vi "Resize Pane.vi"(6 "Pane size":i32, 8 "error in (no error)":errorcluster, 11 "Splitter in":refnum<class "Splitter.lvclass">) -> (0 "error out":errorcluster, 2 "Resized?":bool, 3 "Splitter out":refnum<class "Splitter.lvclass">)   [LabVIEW 2021, in "Splitter.lvclass"]
doc: "Copyright 2018, Wiebe Walstra, wiebe@carya.nl."
uses:
  Splitter.lvclass
  C:/Projects/Dynamic-Scaling/Dynamic Scaling/IContainer/Divider/Divider.lvclass
  Splitter.lvclass/Splitter.ctl
  Divider.lvclass
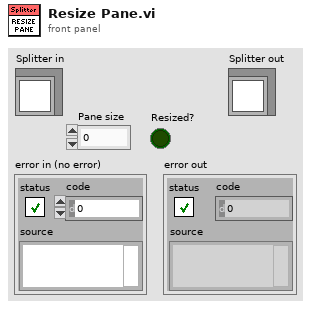
[diagram p1: front panel]
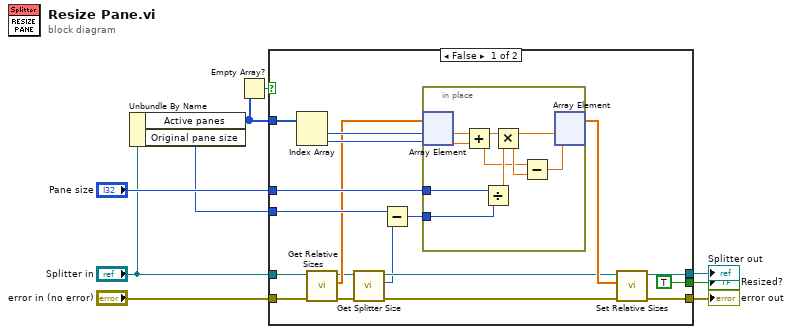
[diagram p0: block diagram]
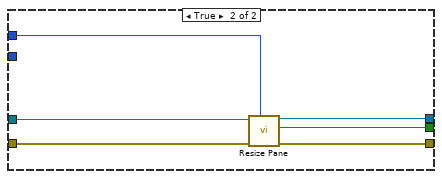
[diagram p2: hidden frame]
diagram:
  n1 = Unbundle By Name("Splitter in") -> ("Active panes"=w2:i32[], "Original pane size"=w1:i16)
  n2 = Empty Array?(array=w2) -> (empty?=w3:bool)
  n3 = case shown="False" w3 {
    tunnel: [w16 w41] -> w9
    tunnel: [TRUE ("Resized?") w40] -> w8
    tunnel: [w14 w39] -> w7
    tunnel: "Pane size" -> [w25 w38]
    tunnel: "error in (no error)" -> [w26 w37]
    tunnel: "Splitter in" -> [w18 w36]
    tunnel: w2 -> [w24 _]
    tunnel: w1 -> [w23 _]
    frame False {
      n4 = Index Array(array=w24) -> (element #1=w22:i32, element #2=w21:i32)  [unwired: 2 in]
      n5 = call "Get Relative Sizes.vi"("error in (no error)"=w26, "Divider in"=w18) -> ("error out"=w19:errorcluster, "Relative sizes"=w17:dbl[], "Divider out"=w12:refnum<class "Splitter.lvclass">)  [unwired: 7 in]
      n6 = call "Get Splitter Size.vi"("error in (no error)"=w19, "Divider in"=w12) -> ("error out"=w13:errorcluster, ".5 Splitter size"=w10:i16, "Divider out"=w11:refnum<class "Splitter.lvclass">)  [unwired: 6 in, 1 out]
      n7 = Subtract(x=w23, y=w10) -> (x-y=w20:i16)
      n8 = in-place {
        in-place-border: w25 -> [w30]
        in-place-border: w20 -> [w29]
        n9 = in-place-array #1(w17, w22, w21) -> (w35:dbl, w34:dbl)
        n10 = Add(x=w35, y=w34) -> (x+y=w28:dbl)
        n11 = Divide(x=w30, y=w29) -> (x/y=w31:dbl)
        n12 = Multiply(x=w28, y=w31) -> (x*y=w33:dbl)
        n13 = Subtract(x=w28, y=w33) -> (x-y=w32:dbl)
        n14 = in-place-array #1(w33, w32) -> (w15:dbl[])  [unwired: 2 out]
      }
      n15 = call "Set Relative Sizes.vi"("error in (no error)"=w13, "Relative sizes"=w15, "Divider in"=w11) -> ("error out"=w16:errorcluster, "Divider out"=w14:refnum<class "Splitter.lvclass">)  [unwired: 7 in]
    }
    frame True {
      n16 = call-parent "Resize Pane.vi"("Pane size"=w38, "error in (no error)"=w37, "IContainer in"=w36) -> ("error out"=w41:errorcluster, "Resized?"=w40:bool, "IContainer out"=w39:refnum<class "Splitter.lvclass">)  [unwired: 6 in]
    }
  }
  "error out" <- w9
  "Splitter out" <- w7
  "Resized?" <- w8
